vi "VNA_CW.vi"(4 "Power (dbm)":dbl=-8.0, 5 "Transport":refnum<class "Transport.lvclass">, 7 "VNA Address":refnum<visa-resource-name>="GPIB0::15::INSTR", 9 "sweep type (0 : linear)":u16(ring)=3 items=["linear sweep", "logarithmic sweep", "frequency list", "CW time sweep", "power sweep"], 10 "sweep time (sec)":dbl=1e-09 format="%.2p", 11 "num points":u16(ring)=8 items=["3", "11", "21 ('20) / 26 ('53)", "51", "101", "201", "401", "801", "1601"]) -> (2 "Polar plot":cluster{dbl[], sgl[]}[](graph))   [LabVIEW 2020]
uses:
  <userlib>/LevyLab/Transport/Transport/Transport.lvclass
  <userlib>/LevyLab/Transport/Transport/Transport.lvclass/Transport.ctl
  <userlib>/LevyLab/Transport/Control Experiment/Control Experiment.lvclass/Control Experiment.ctl
  <userlib>/LevyLab/Transport/Control Experiment/Control Experiment.lvclass
  <instrlib>/Agilent 87XX Series/Agilent 87XX Series.lvlib
  <userlib>/LevyLab/Instrument Framework/Instrument Types/Cryostat/Instrument.Cryostat.lvclass
panel:
  in  "CW freq (Hz)":dbl=704000000.0 format="%.2p"
  out "Data 2":cluster{dbl[], dbl[]}[](graph)
  out "B Field (T)":dbl=0.0003
  out "Temperature (K)":dbl=0.020510017998887152
  in  "Vg (V)":dbl
  in  "Ids (mA)":dbl=9.5
  in  "Vds (V)":dbl=1.3
  in  "Experiment Description":string="B = 0.1T\nVbg(AO6) = 0V\nPower: -35 dBm\nVd: 1.3V\nId: 9.5mA\n"
  in  "Experiment Folder":string="99-test"
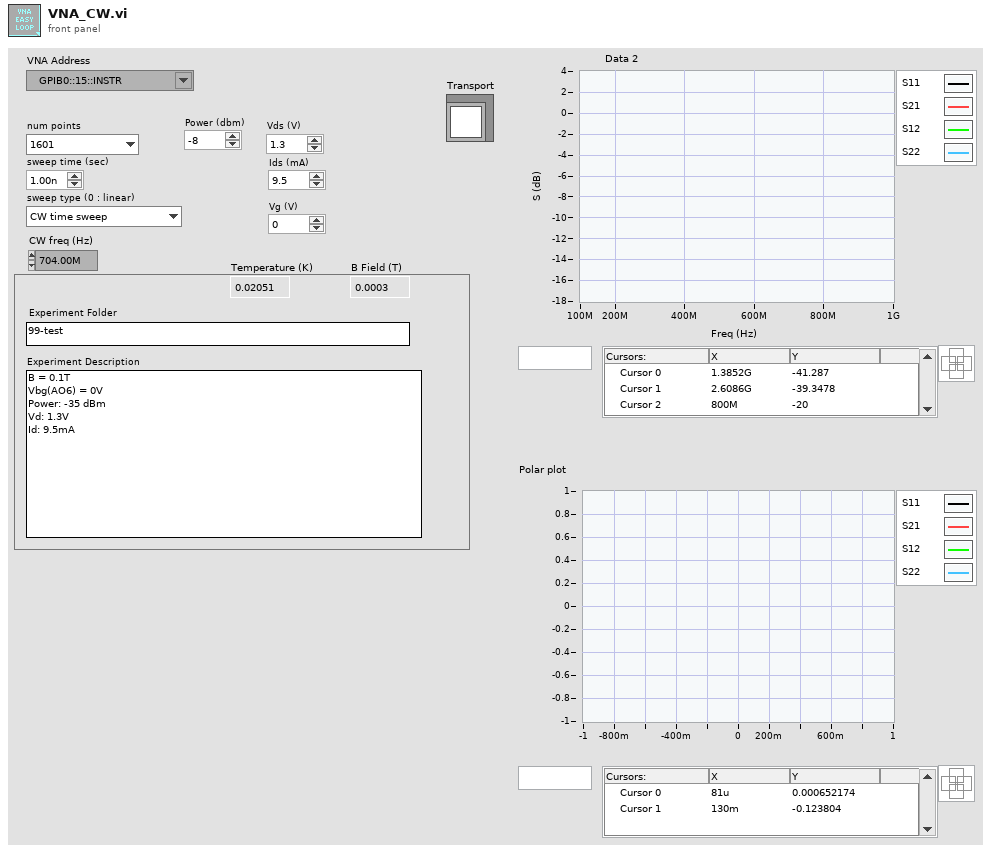
[diagram p1: front panel]
types:
  T1 = enum32{"Bad", "Idle", "Run top level", "Running"}
  T2 = typedef "Control Experiment.lvclass/Instrument Classes--cluster.ctl" = cluster{"DAQ":refnum<class "Instrument.LockinAPI.lvclass">, "Amplifier":refnum<class "Instrument.Amplifier.lvclass">, "Temperature":refnum<class "Instrument.Cryostat.lvclass">, "Magnet":refnum<class "Instrument.Cryostat.lvclass">, "Rotator":refnum<class "Instrument.Cryostat.lvclass">, "Level":refnum<class "Instrument.Cryostat.lvclass">, "Capacitance":refnum<class "Instrument.CBridge.lvclass">, "Delay Line":refnum<class "Instrument.DelayLine.lvclass">, "Strain Cell":refnum<class "Instrument.Strain.lvclass">, "VNA":refnum<class "Instrument.VNA.lvclass">, "Source":refnum<class "Instrument.VSource.lvclass">}
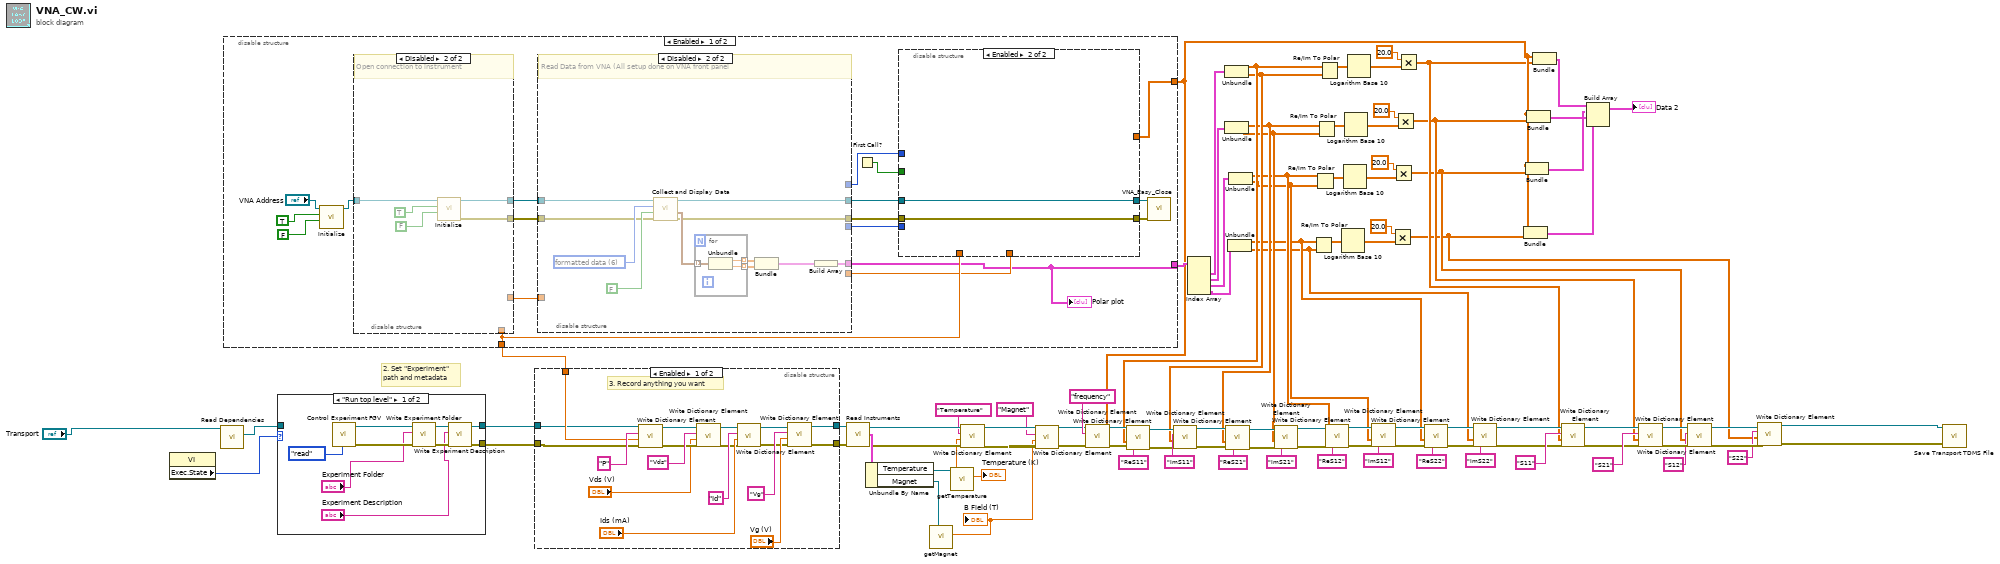
[diagram p0: block diagram]
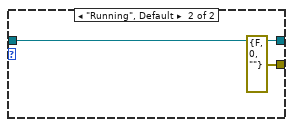
[diagram p2: hidden frame]
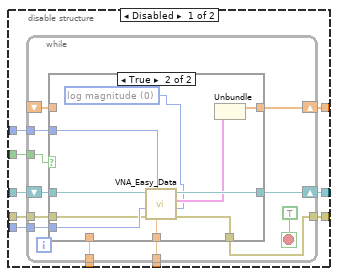
[diagram p4: hidden frame]
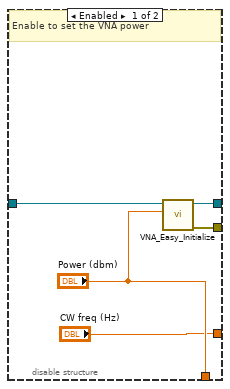
[diagram p6: hidden frame]
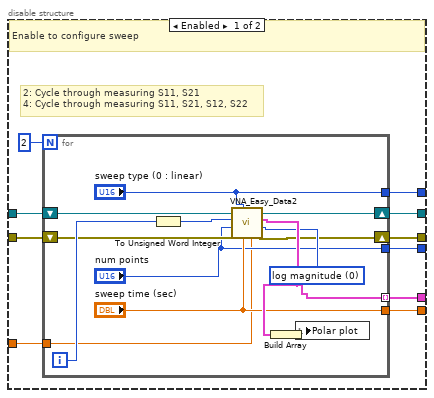
[diagram p7: hidden frame]
diagram:
  # "2. Set \"Experiment\"\npath and metadata"
  n1 = property class="VI"() -> ("Exec.State"=w62:T1)  [unwired: 2 in, 2 out]
  n2 = call <userlib>:"Read Dependencies.vi"("Transport"="Transport") -> ("C.E."=w58:refnum<class "Control Experiment.lvclass">)  [unwired: 8 in, 2 out]
  n3 = disable-structure shown="Enabled" {
    disable-tunnel: [w97 _] -> w57
    disable-tunnel: [w104 _] -> w88
    disable-tunnel: [w105 _] -> w15
    frame Enabled {
      n4 = call <instrlib>:"Initialize.vi"("reset"=FALSE, "ID query"=TRUE, "VISA resource name"="VNA Address") -> ("VISA resource name out"=w108:refnum<visa-resource-name>)  [unwired: 7 in, 1 out]
      n5 = disable-structure shown="Disabled" {
        disable-tunnel: w108 -> [w155 w158]
        disable-tunnel: [w154 w156] -> w113
        disable-tunnel: [w153 w157] -> w112
        disable-tunnel: ["Power (dbm)" _] -> w104
        disable-tunnel: ["CW freq (Hz)" _] -> w96
        frame Enabled {
          # "Enable to set the VNA power"
          n6 = call "VNA_Easy_Initialize.vi"("Power (dbm)"="Power (dbm)", "VISA Refnum in"=w155) -> ("error out"=w153:errorcluster, "VISA Refnum out"=w154:refnum<visa-resource-name>)  [unwired: 8 in]
        }
        frame Disabled {
          # "Open connection to instrument"
          n7 = call <instrlib>:"Initialize.vi"("reset"=FALSE, "ID query"=TRUE, "VISA resource name"=w158) -> ("error out"=w157:errorcluster, "VISA resource name out"=w156:refnum<visa-resource-name>)  [unwired: 7 in]
        }
      }
      n8 = disable-structure shown="Disabled" {
        disable-tunnel: w113 -> [w170 w188]
        disable-tunnel: w112 -> [w169 w189]
        disable-tunnel: [w168 w186] -> w103
        disable-tunnel: [w167 w187] -> w107
        disable-tunnel: [w166 w184] -> w97
        disable-tunnel: [w164 _] -> w101
        disable-tunnel: [w163 _] -> w100
        disable-tunnel: [w162 _] -> w99
        disable-tunnel: w96 -> [w161 _]
        frame Enabled {
          # "2: Cycle through measuring S11, S21\n4: Cycle through measuring S11, S21, S12, S22"
          # "Enable to configure sweep"
          n9 = for {
            N: 2 -> [_]
            tunnel: [w180] -> w166 mode=indexing
            shift-right: [w181] -> w167
            shift-left: w170 -> [w174]
            shift-right: [w178] -> w168
            shift-left: w169 -> [w176]
            tunnel: ["sweep type (0 : linear)"] -> w164
            tunnel: ["sweep time (sec)"] -> w163
            tunnel: ["num points"] -> w162
            tunnel: w161 -> [w171]
            i -> [w183]
            w179 = u16 0 items=["log magnitude", "phase", "delay", "Smith chart", "polar", "linear magnitude", "standing wave ratio", "real", "imaginary"] ("format (0 : log mag)")
            n10 = To Unsigned Word Integer(number=w183) -> (unsigned 16bit integer=w175:u16)
            n11 = call "VNA_Easy_Data2.vi"("format (0 : log mag)"=w179, "CW freq (Hz)"=w171, "sweep time (sec)"="sweep time (sec)", "sweep type (0 : linear)"="sweep type (0 : linear)", "error in (no error)"=w176, "num points"="num points", "measurement (0 : S11)"=w175, "VISA Refnum in"=w174) -> ("error out"=w178:errorcluster, "Data"=w180:cluster{dbl[], sgl[]}, "VISA Refnum out"=w181:refnum<visa-resource-name>)  [unwired: 1 in]
            n12 = Build Array(w180) -> (w182:cluster{dbl[], sgl[]}[])
            n13 = local write "Polar plot"(w182) -> ()
          }
        }
        frame Disabled {
          w194 = u16 6 items=["raw data array 1", "raw data array 2", "raw data array 3", "raw data array 4", "error-corrected data", "error-corrected trace memory", "formatted data", "formatted memory", "formatted data / memory", "formatted data - memory"] ("data type (6 : formatted data)")
          # "Read Data from VNA (All setup done on VNA front panel"
          n14 = call <instrlib>:"Collect and Display Data.vi"("error in (no error)"=w189, "save to file"=FALSE, "data type (6 : formatted data)"=w194, "VISA resource name"=w188) -> ("error out"=w186:errorcluster, "data values"=w191:cluster{"real / stim":dbl, "imag / resp":sgl}[], "VISA resource name out"=w187:refnum<visa-resource-name>)  [unwired: 4 in, 1 out]
          n15 = for {
            tunnel: w191 -> [w197] mode=indexing
            tunnel: [w196] -> w192 mode=indexing
            tunnel: [w195] -> w193 mode=indexing
            n16 = Unbundle(w197) -> ("real / stim"=w196:dbl, "imag / resp"=w195:sgl)
          }
          n17 = Bundle(w192, w193) -> (w185:cluster{dbl[], sgl[]})  [unwired: 1 in]
          n18 = Build Array(w185) -> (w184:cluster{dbl[], sgl[]}[])
        }
      }
      "Polar plot" <- w97
      n19 = First Call?() -> (First Call?: T/F=w98:bool)
      n20 = disable-structure shown="Enabled" {
        disable-tunnel: w107 -> [w123 w150]
        disable-tunnel: [w122 w150] -> w106
        disable-tunnel: [w121 _] -> w105
        disable-tunnel: w104 -> [w120 _]
        disable-tunnel: w103 -> [w119 w149]
        disable-tunnel: [w118 w149] -> w102
        disable-tunnel: w101 -> [w117 _]
        disable-tunnel: w100 -> [w116 _]
        disable-tunnel: w99 -> [w115 _]
        disable-tunnel: w98 -> [w114 _]
        frame Disabled {
          n21 = while {
            shift-right: [w134] -> w122
            shift-left: w123 -> [w135]
            shift-right: [w132] -> w121
            shift-left: _ -> [w131]
            tunnel: w114 -> [w130]
            tunnel: w120 -> [w129]
            tunnel: w119 -> [w128]
            tunnel: [w127] -> w118
            tunnel: w117 -> [w126]
            tunnel: w116 -> [w125]
            tunnel: w115 -> [w124]
            stop <- TRUE stop-if-true
            n22 = case shown="True" w130 {
              tunnel: w135 -> [w137 w140]
              tunnel: [w137 w148] -> w134
              tunnel: [w138 w146] -> w132
              tunnel: w131 -> [w138 _]
              tunnel: w129 -> [_ _]
              tunnel: w128 -> [w136 w139]
              tunnel: [w136 w145] -> w127
              tunnel: w126 -> [_ w144]
              tunnel: w125 -> [_ w143]
              tunnel: w124 -> [_ w142]
              frame False {
              }
              frame True {
                w141 = u16 0 items=["log magnitude", "phase", "delay", "Smith chart", "polar", "linear magnitude", "standing wave ratio", "real", "imaginary"] ("format (0 : log mag)")
                n23 = call "VNA_Easy_Data.vi"("format (0 : log mag)"=w141, "sweep time (sec)"=w143, "sweep type (0 : linear)"=w144, "error in (no error)"=w139, "num points"=w142, "VISA Refnum in"=w140) -> ("error out"=w145:errorcluster, "Data"=w147:cluster{dbl[], sgl[]}, "VISA Refnum out"=w148:refnum<visa-resource-name>)  [unwired: 3 in]
                n24 = Unbundle(w147) -> (w146:dbl[])  [unwired: 1 out]
              }
            }
          }
        }
        frame Enabled {
        }
      }
      n25 = call "VNA_Easy_Close.vi"("error in (no error)"=w102, "VISA Refnum in"=w106) -> ()  [unwired: 9 in, 1 out]
    }
    frame Disabled {
    }
  }
  n26 = case shown="\"Run top level\"" w62 {
    tunnel: [w202 errorcluster {"status"=FALSE, "code"=0, "source"=""} ("error out")] -> w60
    tunnel: [w201 w208] -> w61
    tunnel: w58 -> [_ w208]
    frame "Run top level" {
      n27 = call <userlib>:"Control Experiment FGV.vi"("Function"=enum16{"read", "write"}."read") -> ("error out"=w205:errorcluster, "Control Experiment.lvclass out"=w206:refnum<class "Control Experiment.lvclass">)  [unwired: 9 in]
      n28 = call <userlib>:"Write Experiment Folder.vi"("error in (no error)"=w205, "Experiment Folder"="Experiment Folder", "Control Experiment in"=w206) -> ("error out"=w203:errorcluster, "Control Experiment out"=w204:refnum<class "Control Experiment.lvclass">)  [unwired: 7 in]
      n29 = call <userlib>:"Write Experiment Description.vi"("error in (no error)"=w203, "Experiment Description"="Experiment Description", "Control Experiment in"=w204) -> ("error out"=w202:errorcluster, "Control Experiment out"=w201:refnum<class "Control Experiment.lvclass">)  [unwired: 7 in]
    }
    frame "Running", Default {
    }
  }
  n30 = disable-structure shown="Enabled" {
    disable-tunnel: w61 -> [w218 w228]
    disable-tunnel: w60 -> [w217 w227]
    disable-tunnel: [w223 w228] -> w87
    disable-tunnel: [w209 w227] -> w86
    disable-tunnel: w88 -> [w219 _]
    frame Enabled {
      # "3. Record anything you want"
      n31 = call <userlib>:"Write Dictionary Element.vi"("error in (no error)"=w217, "value"=w219, "key"="P", "Control Experiment in"=w218) -> ("error out"=w215:errorcluster, "Control Experiment out"=w216:refnum<class "Control Experiment.lvclass">)  [unwired: 6 in]
      n32 = call <userlib>:"Write Dictionary Element.vi"("error in (no error)"=w215, "value"="Vds (V)", "key"="Vds", "Control Experiment in"=w216) -> ("error out"=w212:errorcluster, "Control Experiment out"=w225:refnum<class "Control Experiment.lvclass">)  [unwired: 6 in]
      n33 = call <userlib>:"Write Dictionary Element.vi"("error in (no error)"=w212, "value"="Ids (mA)", "key"="Id", "Control Experiment in"=w225) -> ("error out"=w210:errorcluster, "Control Experiment out"=w224:refnum<class "Control Experiment.lvclass">)  [unwired: 6 in]
      n34 = call <userlib>:"Write Dictionary Element.vi"("error in (no error)"=w210, "value"="Vg (V)", "key"="Vg", "Control Experiment in"=w224) -> ("error out"=w209:errorcluster, "Control Experiment out"=w223:refnum<class "Control Experiment.lvclass">)  [unwired: 6 in]
    }
    frame Disabled {
    }
  }
  n35 = call <userlib>:"Read Instruments.vi"("error in (no error)"=w86, "Control Experiment in"=w87) -> ("error out"=w82:errorcluster, "Instruments"=w85:T2, "Control Experiment out"=w81:refnum<class "Control Experiment.lvclass">)  [unwired: 7 in]
  n36 = Unbundle By Name(w85) -> ("Temperature"=w83:refnum<class "Instrument.Cryostat.lvclass">, "Magnet"=w84:refnum<class "Instrument.Cryostat.lvclass">)
  n37 = call-dynamic "getMagnet.vi"("Instrument.Cryostat in"=w84) -> ("B Field (T)"=w73:dbl)  [unwired: 6 in, 4 out]
  "B Field (T)" <- w73
  n38 = call-dynamic "getTemperature.vi"("Instrument.Cryostat in"=w83) -> ("Temperature (K)"=w80:dbl)  [unwired: 6 in, 4 out]
  "Temperature (K)" <- w80
  n39 = call <userlib>:"Write Dictionary Element.vi"("error in (no error)"=w82, "value"=w80, "key"="Temperature", "Control Experiment in"=w81) -> ("error out"=w75:errorcluster, "Control Experiment out"=w78:refnum<class "Control Experiment.lvclass">)  [unwired: 6 in]
  n40 = call <userlib>:"Write Dictionary Element.vi"("error in (no error)"=w75, "value"=w73, "key"="Magnet", "Control Experiment in"=w78) -> ("error out"=w76:errorcluster, "Control Experiment out"=w77:refnum<class "Control Experiment.lvclass">)  [unwired: 6 in]
  n41 = call <userlib>:"Write Dictionary Element.vi"("error in (no error)"=w76, "value"=w15, "key"="frequency", "Control Experiment in"=w77) -> ("error out"=w47:errorcluster, "Control Experiment out"=w49:refnum<class "Control Experiment.lvclass">)  [unwired: 6 in]
  n42 = Index Array(array=w57) -> (element #1=w95:cluster{dbl[], sgl[]}, element #2=w89:cluster{dbl[], sgl[]}, element #3=w65:cluster{dbl[], sgl[]}, element #4=w63:cluster{dbl[], sgl[]})  [unwired: 4 in]
  n43 = Unbundle(w95) -> (w25:dbl[], w24:sgl[])
  n44 = call <userlib>:"Write Dictionary Element.vi"("error in (no error)"=w47, "value"=w25, "key"="ReS11", "Control Experiment in"=w49) -> ("error out"=w46:errorcluster, "Control Experiment out"=w48:refnum<class "Control Experiment.lvclass">)  [unwired: 6 in]
  n45 = call <userlib>:"Write Dictionary Element.vi"("error in (no error)"=w46, "value"=w24, "key"="ImS11", "Control Experiment in"=w48) -> ("error out"=w41:errorcluster, "Control Experiment out"=w43:refnum<class "Control Experiment.lvclass">)  [unwired: 6 in]
  n46 = Unbundle(w89) -> (w11:dbl[], w10:sgl[])
  n47 = call <userlib>:"Write Dictionary Element.vi"("error in (no error)"=w41, "value"=w11, "key"="ReS21", "Control Experiment in"=w43) -> ("error out"=w40:errorcluster, "Control Experiment out"=w42:refnum<class "Control Experiment.lvclass">)  [unwired: 6 in]
  n48 = Unbundle(w63) -> (w7:dbl[], w6:sgl[])
  n49 = Unbundle(w65) -> (w9:dbl[], w8:sgl[])
  n50 = call <userlib>:"Write Dictionary Element.vi"("error in (no error)"=w40, "value"=w10, "key"="ImS21", "Control Experiment in"=w42) -> ("error out"=w28:errorcluster, "Control Experiment out"=w29:refnum<class "Control Experiment.lvclass">)  [unwired: 6 in]
  n51 = Re/Im To Polar(2:w6, 3:w7) -> (1:w17:dbl[])  [unwired: 1 out]
  n52 = Re/Im To Polar(2:w8, 3:w9) -> (1:w20:dbl[])  [unwired: 1 out]
  n53 = Re/Im To Polar(2:w10, 3:w11) -> (1:w1:dbl[])  [unwired: 1 out]
  n54 = Re/Im To Polar(2:w24, 3:w25) -> (1:w53:dbl[])  [unwired: 1 out]
  n55 = call <userlib>:"Write Dictionary Element.vi"("error in (no error)"=w28, "value"=w9, "key"="ReS12", "Control Experiment in"=w29) -> ("error out"=w36:errorcluster, "Control Experiment out"=w37:refnum<class "Control Experiment.lvclass">)  [unwired: 6 in]
  n56 = Logarithm Base 10(1:w17) -> (0:w16:dbl[])
  n57 = Logarithm Base 10(1:w20) -> (0:w19:dbl[])
  n58 = Logarithm Base 10(1:w1) -> (0:w22:dbl[])
  n59 = Logarithm Base 10(1:w53) -> (0:w52:dbl[])
  n60 = call <userlib>:"Write Dictionary Element.vi"("error in (no error)"=w36, "value"=w8, "key"="ImS12", "Control Experiment in"=w37) -> ("error out"=w31:errorcluster, "Control Experiment out"=w33:refnum<class "Control Experiment.lvclass">)  [unwired: 6 in]
  n61 = Multiply(x=20.0, y=w16) -> (x*y=w2:dbl[])
  n62 = Multiply(x=20.0, y=w19) -> (x*y=w3:dbl[])
  n63 = Multiply(x=20.0, y=w22) -> (x*y=w4:dbl[])
  n64 = Multiply(x=20.0, y=w52) -> (x*y=w5:dbl[])
  n65 = call <userlib>:"Write Dictionary Element.vi"("error in (no error)"=w31, "value"=w7, "key"="ReS22", "Control Experiment in"=w33) -> ("error out"=w30:errorcluster, "Control Experiment out"=w32:refnum<class "Control Experiment.lvclass">)  [unwired: 6 in]
  n66 = call <userlib>:"Write Dictionary Element.vi"("error in (no error)"=w30, "value"=w6, "key"="ImS22", "Control Experiment in"=w32) -> ("error out"=w26:errorcluster, "Control Experiment out"=w27:refnum<class "Control Experiment.lvclass">)  [unwired: 6 in]
  n67 = Bundle(w15, w2) -> (w12:cluster{dbl[], dbl[]})  [unwired: 1 in]
  n68 = Bundle(w15, w3) -> (w13:cluster{dbl[], dbl[]})  [unwired: 1 in]
  n69 = Bundle(w15, w4) -> (w14:cluster{dbl[], dbl[]})  [unwired: 1 in]
  n70 = Bundle(w15, w5) -> (w56:cluster{dbl[], dbl[]})  [unwired: 1 in]
  n71 = call <userlib>:"Write Dictionary Element.vi"("error in (no error)"=w26, "value"=w5, "key"="S11", "Control Experiment in"=w27) -> ("error out"=w91:errorcluster, "Control Experiment out"=w90:refnum<class "Control Experiment.lvclass">)  [unwired: 6 in]
  n72 = Build Array(w56, w14, w13, w12) -> (→"Data 2":cluster{dbl[], dbl[]}[])
  n73 = call <userlib>:"Write Dictionary Element.vi"("error in (no error)"=w91, "value"=w4, "key"="S21", "Control Experiment in"=w90) -> ("error out"=w69:errorcluster, "Control Experiment out"=w72:refnum<class "Control Experiment.lvclass">)  [unwired: 6 in]
  n74 = call <userlib>:"Write Dictionary Element.vi"("error in (no error)"=w69, "value"=w3, "key"="S12", "Control Experiment in"=w72) -> ("error out"=w68:errorcluster, "Control Experiment out"=w71:refnum<class "Control Experiment.lvclass">)  [unwired: 6 in]
  n75 = call <userlib>:"Write Dictionary Element.vi"("error in (no error)"=w68, "value"=w2, "key"="S22", "Control Experiment in"=w71) -> ("error out"=w64:errorcluster, "Control Experiment out"=w70:refnum<class "Control Experiment.lvclass">)  [unwired: 6 in]
  n76 = call <userlib>:"Save Transport TDMS File.vi"("error in (no error)"=w64, "Control Experiment in"=w70) -> ()  [unwired: 8 in, 2 out]
